vi "Initialize.vi"(8 "error in (no error)":errorcluster, 9 "transceiver settings":T1, 10 "Transfer Groups Configurations":T2[](array[typedef]) {"Transfers"."channel configurations"."buffer offset" format="%d bytes"}, 11 "DSFPlugin in":refnum<class "DSFPlugin Transceiver.lvclass">) -> (0 "error out":errorcluster, 3 "DSFPlugin out":refnum<class "DSFPlugin Transceiver.lvclass">)   [LabVIEW 2017, in "DSFPluginTest.lvlib" / "DSFPlugin Transceiver.lvclass"]
uses:
  DSFPlugin Transceiver.lvclass
  builds/Data Sharing Framework/Current/Data Sharing Framework Core/DSF Core.lvlibp/Configuration/Public/Controls/DSF Engine Transfer Group Configuration.ctl
  builds/Data Sharing Framework/Current/Data Sharing Framework Core/DSF Core.lvlibp/Configuration/Public/Controls/DSF Direction.ctl
  builds/Data Sharing Framework/Current/Data Sharing Framework Core/DSF Core.lvlibp/Configuration/Public/Controls/DSF Timing Info.ctl
  builds/Data Sharing Framework/Current/Data Sharing Framework Core/DSF Core.lvlibp/Configuration/Public/Controls/DSF Engine Transfer Configuration.ctl
  builds/Data Sharing Framework/Current/Data Sharing Framework Core/DSF Core.lvlibp/Configuration/Public/Controls/DSF Byte Order.ctl
  builds/Data Sharing Framework/Current/Data Sharing Framework Core/DSF Core.lvlibp/Configuration/Public/Controls/DSF Engine Channel Configuration.ctl
  builds/Data Sharing Framework/Current/Data Sharing Framework Core/DSF Core.lvlibp/Configuration/Public/Controls/DSF Data Type.ctl
  builds/Data Sharing Framework/Current/Data Sharing Framework Core/DSF Core.lvlibp/Configuration/Public/Controls/DSF Settings Info.ctl
  DSFPlugin Transceiver.lvclass/DSFPlugin Transceiver.ctl
  builds/Data Sharing Framework/Current/Data Sharing Framework Core/DSF Core.lvlibp
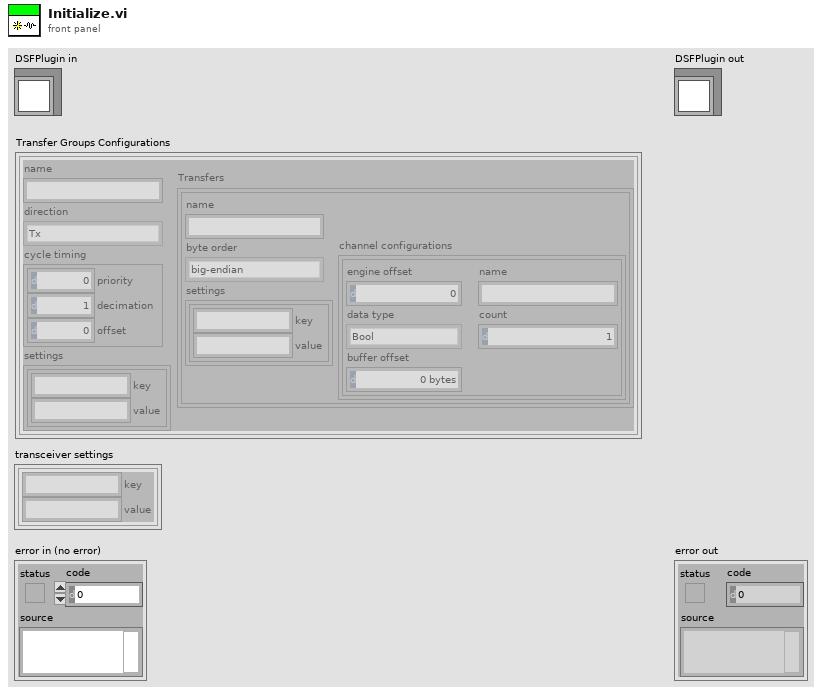
[diagram p1: front panel]
types:
  T1 = typedef "DSF Core.lvlibp/DSF Settings Info.ctl" = cluster{"key":string, "value":string}[]
  T2 = typedef "DSF Core.lvlibp/DSF Engine Transfer Group Configuration.ctl" = cluster{"name":string, "direction":T3, "cycle timing":T4, "Transfers":T5[], "settings":T1}
  T3 = typedef "DSF Core.lvlibp/DSF Direction.ctl" = enum8{"Tx", "Rx"}
  T4 = typedef "DSF Core.lvlibp/DSF Timing Info.ctl" = cluster{"priority":u64, "decimation":u64, "offset":u64}
  T5 = typedef "DSF Core.lvlibp/DSF Engine Transfer Configuration.ctl" = cluster{"name":string, "byte order":T6, "channel configurations":T7[], "settings":T1}
  T6 = typedef "DSF Core.lvlibp/DSF Byte Order.ctl" = enum8{"big-endian", "little-endian"}
  T7 = typedef "DSF Core.lvlibp/DSF Engine Channel Configuration.ctl" = cluster{"engine offset":u64, "name":string, "data type":T8, "count":u64, "buffer offset":u64}
  T8 = typedef "DSF Core.lvlibp/DSF Data Type.ctl" = enum8{"Bool", "SGL", "DBL", "I8", "I16", "I32", "I64", "U8", "U16", "U32", "U64"}
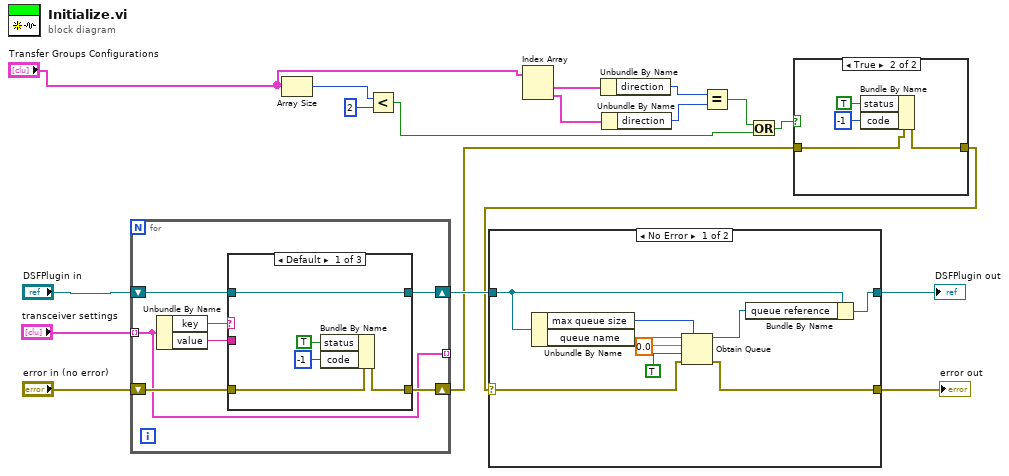
[diagram p0: block diagram]
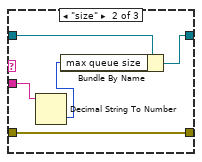
[diagram p4: hidden frame]
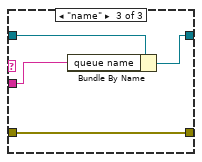
[diagram p5: hidden frame]
diagram:
  n1 = for {
    tunnel: "transceiver settings" -> [w19] mode=indexing
    shift-right: [w22] -> w17
    shift-left: "DSFPlugin in" -> [w23]
    shift-right: [w20] -> w7
    shift-left: "error in (no error)" -> [w21]
    tunnel: [w19] -> _ mode=indexing
    n2 = Unbundle By Name(w19) -> ("key"=w25:string, "value"=w24:string)
    n3 = case shown="Default" w25 {
      tunnel: w24 -> [_ w33 w36]
      tunnel: w23 -> [w30 w35 w39]
      tunnel: [w30 w34 w38] -> w22
      tunnel: w21 -> [w29 w31 w37]
      tunnel: [w28 w31 w37] -> w20
      frame Default {
        n4 = Bundle By Name(cluster=w29, "status"=TRUE, "code"=-1) -> (w28:errorcluster)
      }
      frame "size" {
        n5 = Decimal String To Number(string=w33) -> (number=w32:i32)  [unwired: 2 in, 1 out]
        n6 = Bundle By Name(cluster=w35, "max queue size"=w32) -> (w34:refnum<class "DSFPlugin Transceiver.lvclass">)
      }
      frame "name" {
        n7 = Bundle By Name(cluster=w39, "queue name"=w36) -> (w38:refnum<class "DSFPlugin Transceiver.lvclass">)
      }
    }
  }
  n8 = Array Size(array="Transfer Groups Configurations") -> (size(s)=w15:i32)
  n9 = Less?(x=w15, y=2) -> (x < y?=w8:bool)
  n10 = Index Array(array="Transfer Groups Configurations") -> (element #1=w13:T2, element #2=w12:T2)  [unwired: 2 in]
  n11 = Unbundle By Name(w13) -> ("direction"=w10:T3)
  n12 = Unbundle By Name(w12) -> ("direction"=w11:T3)
  n13 = Equal?(x=w10, y=w11) -> (x = y?=w9:bool)
  n14 = Or(x=w9, y=w8) -> (x .or. y?=w5:bool)
  n15 = case shown="True" w5 {
    tunnel: w7 -> [w40 w42]
    tunnel: [w40 w41] -> w6
    frame False {
    }
    frame True {
      n16 = Bundle By Name(cluster=w42, "status"=TRUE, "code"=-1) -> (w41:errorcluster)
    }
  }
  n17 = case shown="No Error" w6 {
    selector: w6 -> [w45 w54]
    tunnel: [w49 w55] -> w18
    tunnel: w17 -> [w47 w55]
    tunnel: [w46 w54] -> w16
    frame No Error {
      n18 = Unbundle By Name(w47) -> ("max queue size"=w52:i32, "queue name"=w53:string)
      n19 = Obtain Queue(max queue size (-1, unlimited)=w52, name (unnamed)=w53, element data type=0.0, create if not found? (T)=TRUE, error in (no error)=w45) -> (queue out=w48:refnum<queue>, error out=w46:errorcluster)  [unwired: 1 out]
      n20 = Bundle By Name(cluster=w47, "queue reference"=w48) -> (w49:refnum<class "DSFPlugin Transceiver.lvclass">)
    }
    frame Error {
    }
  }
  "DSFPlugin out" <- w18
  "error out" <- w16
